vi "Create Channel Arbitrary Waveform I16 [ACH].vi"(8 "error in (no error)":errorcluster, 9 "Waveform Data Array":i16[](array[numeric]) caption="waveform data array", 10 "Channel Name (\"\")":string="CHANNEL1" caption="channel name (\"CHANNEL1\")", 11 "CS++Fgen in":refnum<class "CS++Fgen.lvclass">) -> (0 "error out":errorcluster, 2 "waveform handle":i32, 3 "CS++Fgen out":refnum<class "CS++Fgen.lvclass">)   [LabVIEW 2013, in "CS++Fgen.lvlib" / "CS++Fgen.lvclass"]
doc: "This VI creates a channel-specific arbitrary waveform and returns a handle that identifies that waveform. Data is passed in as 16-bit binary data. If the arbitrary waveform generator supports formats smaller than 16 bits, read the IviFgen Binary Alignment [AB] property to determine whether to left or right justify the data before passing it to this call. \n\nYou pass this handle to the IviFgen Configure Arbitrary Waveform [ARB] VI to produce that waveform. You also use the handles this VI returns to specify a sequence of arbitrary waveforms with the IviFgen Create Arbitrary Sequence [SEQ] VI.\n\nIf the instrument does not support channel-based arbitrary waveform creation, use the IviFgen Create Arbitrary Waveform [ARB] VI.\n\nUse the IviFgen Create Channel Arbitrary Waveform Int32 [AB] VI to create a channel-specific arbitrary waveform if you want to pass data in 32-bit binary. Use the IviFgen Create Channel Arbitrary Waveform [ACH] VI to create a channel-specific arbitrary waveform with normalized data.\n\nNote:\n\n(1) This VI is part of the IviFgenArbWfmBinary [AB] extension group."
uses:
  CS++Fgen.lvclass
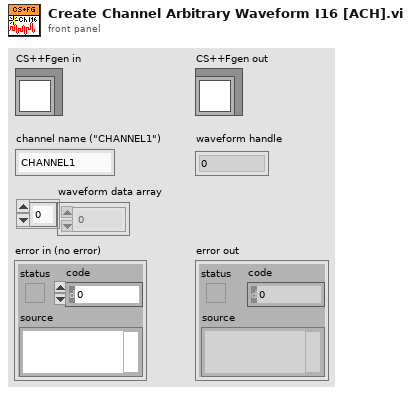
[diagram p1: front panel]
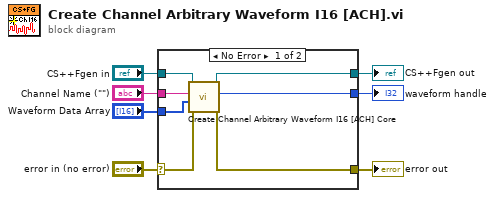
[diagram p0: block diagram]
diagram:
  n1 = case shown="No Error" "error in (no error)" {
    selector: "error in (no error)" -> [w11 w16]
    tunnel: [w10 w16] -> w6
    tunnel: [w12 w15] -> w4
    tunnel: "CS++Fgen in" -> [w13 w15]
    tunnel: "Waveform Data Array" -> [w9 _]
    tunnel: "Channel Name (\"\")" -> [w14 _]
    tunnel: [w8 _] -> w1
    frame No Error {
      n2 = call-dynamic "Create Channel Arbitrary Waveform I16 [ACH] Core.vi"("error in (no error)"=w11, "Waveform Data Array"=w9, "Channel Name (\"\")"=w14, "CS++Fgen in"=w13) -> ("error out"=w10:errorcluster, "waveform handle"=w8:i32, "CS++Fgen out"=w12:refnum<class "CS++Fgen.lvclass">)  [unwired: 5 in]
    }
    frame Error {
    }
  }
  "error out" <- w6
  "CS++Fgen out" <- w4
  "waveform handle" <- w1
